vi "mongo_check_is_master.vi"(8 "error in (no error)":errorcluster, 11 "conn in":T1) -> (0 "error out":errorcluster, 3 "conn out":T1)   [LabVIEW 2013]
uses:
  mongo.ctl
panel:
  in  "bson_iterator":i32
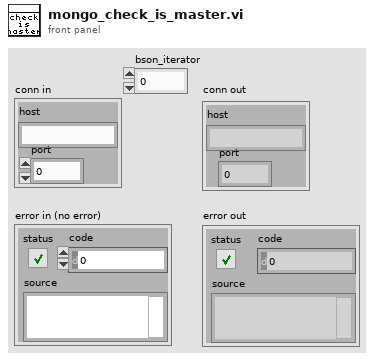
[diagram p1: front panel]
types:
  T1 = typedef "mongo.ctl" = cluster{"host":string, "port":i32}
  T2 = typedef "bson.ctl" = cluster{i32}
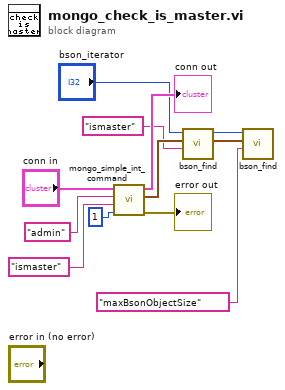
[diagram p0: block diagram]
diagram:
  n1 = call "mongo_simple_int_command.vi"("arg"=1, "cmdstr"="ismaster", "db"="admin", "conn in"="conn in") -> ("result"=→"error out":errorcluster, "out"=w6:T2, "conn out"=→"conn out":T1)  [unwired: 5 in]
  n2 = call "bson_find.vi"("name"="ismaster", "obj in"=w6, "bson_iterator"="bson_iterator") -> ("obj out"=w3:T2, "bson_iterator out"=w1:i32)  [unwired: 7 in]
  n3 = call "bson_find.vi"("name"="maxBsonObjectSize", "obj in"=w3, "bson_iterator"=w1) -> ()  [unwired: 7 in, 2 out]
